vi "SetContinousMode.vi"(8 "error in (no error)":errorcluster, 10 "Cont Acquisition":bool, 11 "ScopeBase In":refnum<class "ScopeBase.lvclass">) -> (0 "error out":errorcluster, 3 "ScopeBase Out":refnum<class "ScopeBase.lvclass">)   [LabVIEW 2018, in "ScopeBase.lvclass"]
uses:
  ScopeBase.lvclass
  ScopeBase.lvclass/ScopeBase.ctl
  <vilib>/Utility/error.llb/Error Cluster From Error Code.vi
  <vilib>/rvi/errors/niLvFpgaAdjustHostInterfaceError.vi
  <vilib>/rvi/interface/nirviReadWriteControl/nirviReadWriteControl.xnode
  FpgaRef/FpgaRefBase/Common FPGA ref.ctl
  FpgaRef/FpgaRefBase/FpgaRefBase.lvclass
  NiFpgaLv.dll
  <vilib>/rvi/interface/Simulation/niFpgaSimulationCallBeginRW.vi
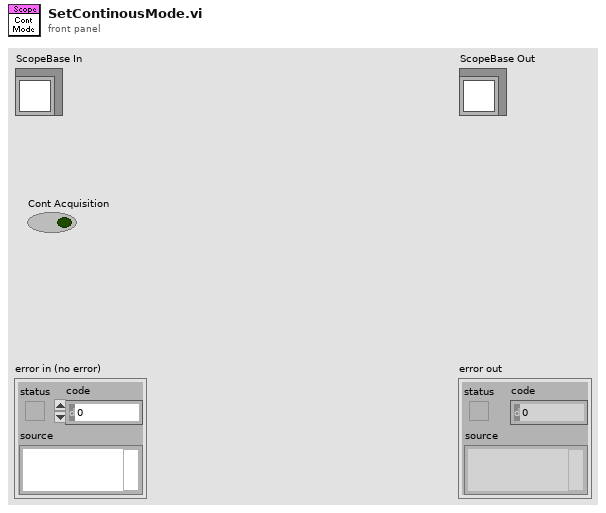
[diagram p1: front panel]
types:
  T1 = typedef "Common FPGA ref.ctl" = refnum<k20>
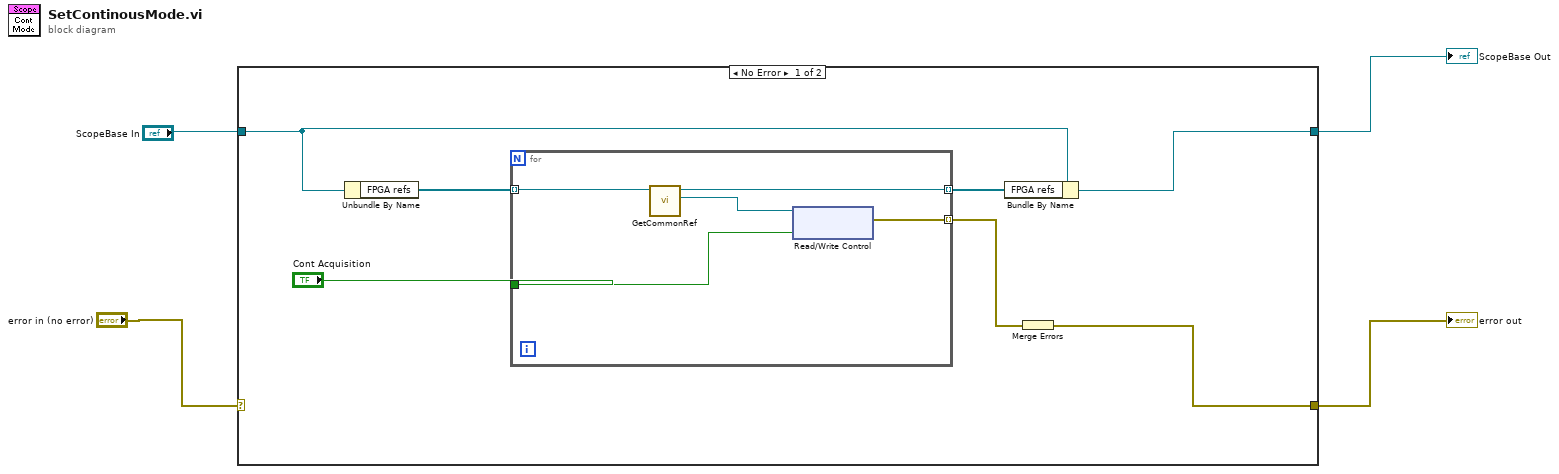
[diagram p0: block diagram]
diagram:
  n1 = case shown="No Error" "error in (no error)" {
    selector: "error in (no error)" -> [_ w18]
    tunnel: [w5 w18] -> w1
    tunnel: [w9 w17] -> w2
    tunnel: "ScopeBase In" -> [w7 w17]
    frame No Error {
      n2 = Unbundle By Name(w7) -> ("FPGA refs"=w11:refnum<class "FpgaRefBase.lvclass">[])
      n3 = for {
        tunnel: "Cont Acquisition" -> [w13]
        tunnel: w11 -> [w16] mode=indexing
        tunnel: [w15] -> w10 mode=indexing
        tunnel: [w12] -> w6 mode=indexing
        n4 = call-dynamic "GetCommonRef.vi"("FpgaRefBase in"=w16) -> ("Common ref"=w14:T1, "FpgaRefBase out"=w15:refnum<class "FpgaRefBase.lvclass">)  [unwired: 8 in, 1 out]
        n5 = xnode "Read/Write Control"("FPGA VI Reference In"=w14, "Continuous"=w13) -> ("error out"=w12:errorcluster)  [unwired: 1 in, 1 out]
      }
      n6 = Bundle By Name(cluster=w7, "FPGA refs"=w10) -> (w9:refnum<class "ScopeBase.lvclass">)
      n7 = Merge Errors(w6) -> (w5:errorcluster)
    }
    frame Error {
    }
  }
  "error out" <- w1
  "ScopeBase Out" <- w2
